vi "Serialize.vi"(7 "DestinationFolder":path, 8 "error in":errorcluster, 9 "OwningElement in":refnum<k20>, 10 "Document in":refnum<k20>, 11 "DocumentType in":refnum<class "Document.lvclass">) -> (0 "error out":errorcluster, 1 "OwningElement out":refnum<k20>, 2 "Document out":refnum<k20>, 3 "DocumentType out":refnum<class "Document.lvclass">)   [LabVIEW 2021, in "ProligentXMLGenerator.lvlib" / "Document.lvclass"]
uses:
  Document.lvclass
  Document.lvclass/Document.ctl
  Base/DOMSupport/DOMSupport.lvlib
  <vilib>/xml/NI_XML.lvlib
  CustomData/CustomData.lvclass
  <vilib>/xml/Close Reference(Node).vi
  Base/Guid/Guid.lvclass
  C:/Projects/proligent-xml-generator-labview/src/ProligentXMLGenerator/Base/NonEmptyString/NonEmptyString.lvclass
  C:/Projects/proligent-xml-generator-labview/src/ProligentXMLGenerator/Base/String/String.lvclass
  C:/Projects/proligent-xml-generator-labview/src/ProligentXMLGenerator/Base/Attribute/Attribute.lvclass
  C:/Projects/proligent-xml-generator-labview/src/ProligentXMLGenerator/Base/Guid/Guid.lvclass
  Base/NonEmptyString_255/NonEmptyString_255.lvclass
  C:/Projects/proligent-xml-generator-labview/src/ProligentXMLGenerator/Base/NonEmptyString_255/NonEmptyString_255.lvclass
  Base/NonNullableString_600/NonNullableString_600.lvclass
  C:/Projects/proligent-xml-generator-labview/src/ProligentXMLGenerator/Base/NonNullableString/NonNullableString.lvclass
  C:/Projects/proligent-xml-generator-labview/src/ProligentXMLGenerator/Base/NonNullableString_600/NonNullableString_600.lvclass
  Base/String/String.lvclass
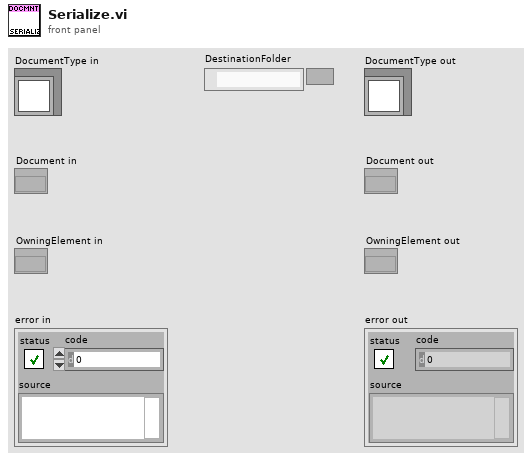
[diagram p1: front panel]
types:
  T1 = typedef "ProligentXMLGenerator.lvlib/Document.lvclass/Data.ctl" = cluster{"Name":string, "CustomData":refnum<class "CustomData.lvclass">, "Identifier":refnum<class "Guid.lvclass">, "NameType":refnum<class "NonEmptyString_255.lvclass">, "FileName":refnum<class "NonEmptyString_255.lvclass">, "Description":refnum<class "NonNullableString_600.lvclass">, "FilePath":path, "DestinationFolder":path}
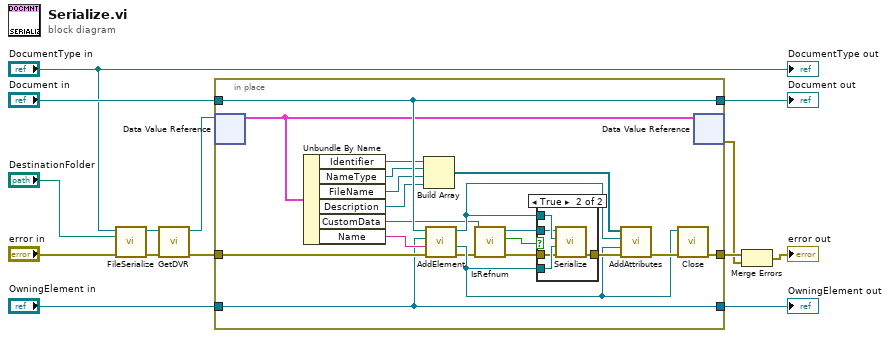
[diagram p0: block diagram]
diagram:
  n1 = call "FileSerialize.vi"("error in (no error)"="error in", "DestinationFolder"="DestinationFolder", "DocumentType in"="DocumentType in") -> ("error out"=w4:errorcluster, "DocumentType out"=w2:refnum<class "Document.lvclass">)  [unwired: 7 in]
  n2 = call "GetDVR.vi"("error in"=w4, "Document in"=w2) -> ("error out"=w8:errorcluster, "DVRReference"=w7:refnum<data-value>)  [unwired: 8 in]
  n3 = in-place "In Place Element Structure" {
    in-place-border: [w32] -> w9
    in-place-border: "Document in" -> [w31]
    in-place-border: w8 -> [w34]
    in-place-border: "OwningElement in" -> [w30]
    in-place-border: [w31] -> w11
    in-place-border: [w30] -> w10
    n4 = in-place-dvr #1(w7) -> (w29:T1)  [unwired: 1 out]
    n5 = Unbundle By Name(w29) -> ("Identifier"=w25:refnum<class "Guid.lvclass">, "NameType"=w24:refnum<class "NonEmptyString_255.lvclass">, "FileName"=w23:refnum<class "NonEmptyString_255.lvclass">, "Description"=w22:refnum<class "NonNullableString_600.lvclass">, "CustomData"=w17:refnum<class "CustomData.lvclass">, "Name"=w33:string)
    n6 = Build Array(w25, w24, w23, w22) -> (w21:refnum<class "String.lvclass">[])
    n7 = call "AddElement.vi"("error in"=w34, "Name"=w33, "OwningElement in"=w30, "Document in"=w31) -> ("error out"=w20:errorcluster, "NewElement"=w26:refnum<k20>, "Document out"=w18:refnum<k20>)  [unwired: 4 in, 1 out]
    n8 = call "IsRefnum.vi"("error in"=w20, "CustomDataType in"=w17) -> ("error out"=w19:errorcluster, "IsRefnum"=w15:bool, "CustomDataType out"=w16:refnum<class "CustomData.lvclass">)  [unwired: 7 in]
    n9 = case shown="True" w15 {
      tunnel: [w35 w40] -> w28
      tunnel: w26 -> [_ w39]
      tunnel: w19 -> [w35 w38]
      tunnel: w18 -> [_ w37]
      tunnel: w16 -> [_ w36]
      frame False {
      }
      frame True {
        n10 = call "Serialize.vi"("error in"=w38, "OwningElement in"=w39, "Document in"=w37, "CustomDataType in"=w36) -> ("error out"=w40:errorcluster)  [unwired: 4 in, 3 out]
      }
    }
    n11 = call "AddAttributes.vi"("error in"=w28, "OwningElement in"=w26, "Document in"=w18, "Attributes"=w21) -> ("error out"=w27:errorcluster)  [unwired: 5 in, 2 out]
    n12 = call-poly <vilib>:"Close.vi"("error in (no error)"=w27, "node"=w26) -> ("error out"=w32:errorcluster)  [unwired: 7 in]
    n13 = in-place-dvr #1(w29) -> (w6:errorcluster)  [unwired: 1 out]
  }
  "OwningElement out" <- w10
  "Document out" <- w11
  n14 = Merge Errors(w9, w6) -> (→"error out":errorcluster)
  "DocumentType out" <- "DocumentType in"
